vi "纳清_温度校准.vi"(7 "探头":T1(ring), 8 "error in (no error)":errorcluster caption="错误输入（无错误）", 10 "校准温度":sgl, 11 "MB session in":refnum<class "MB_Master.lvclass">) -> (0 "error out":errorcluster caption="错误输出", 3 "MB session out":refnum<class "MB_Master.lvclass">)   [LabVIEW 2016, in "斯坦道多参数.lvlib"]
uses:
  <vilib>/Plasmionique/MB Master/MB_Master/MB_Master.lvclass
  <vilib>/Plasmionique/MB Master/MB Master.lvlib
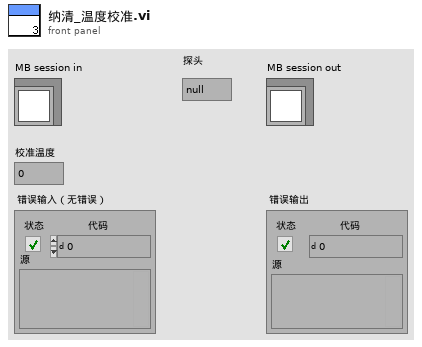
[diagram p1: front panel]
types:
  T1 = enum16{"null", "pH", "DO", "浊度", "电导率", "叶绿素a", "藻密度", "氨氮"}
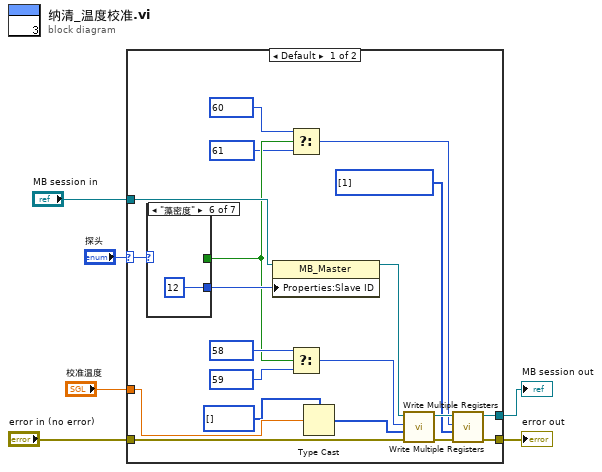
[diagram p0: block diagram]
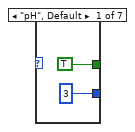
[diagram p2: hidden frame]
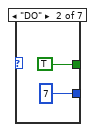
[diagram p3: hidden frame]
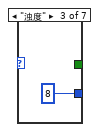
[diagram p4: hidden frame]
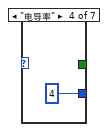
[diagram p5: hidden frame]
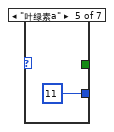
[diagram p6: hidden frame]
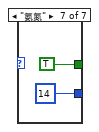
[diagram p7: hidden frame]
diagram:
  n1 = case shown="Default" "探头" {
    selector: "探头" -> [w20 _]
    tunnel: "error in (no error)" -> [w26 w37]
    tunnel: [w17 w37] -> w5
    tunnel: "MB session in" -> [w24 w38]
    tunnel: [w15 w38] -> w3
    tunnel: "校准温度" -> [w22 _]
    frame Default {
      n2 = case shown="\"藻密度\"" w20 {
        tunnel: [3 7 8 4 11 12 14] -> w23
        tunnel: [TRUE TRUE _ _ _ _ TRUE] -> w10
        frame "pH", Default {
        }
        frame "DO" {
        }
        frame "浊度" {
        }
        frame "电导率" {
        }
        frame "叶绿素a" {
        }
        frame "藻密度" {
        }
        frame "氨氮" {
        }
      }
      n3 = property class="MB_Master"(reference=w24, "Properties:Slave ID"=w23) -> (reference out=w25:refnum<class "MB_Master.lvclass">)  [unwired: 1 in, 1 out]
      n4 = Select(t=u16 60 ("starting address"), s=w10, f=u16 61 ("starting address")) -> (s? t:f=w7:u16)
      n5 = Select(t=u16 58 ("starting address"), s=w10, f=u16 59 ("starting address")) -> (s? t:f=w11:u16)
      n6 = Type Cast(type=u16[] [], x=w22) -> (*(type *) &x=w21:u16[])
      n7 = call <vilib>:"Write Multiple Registers.vi"("error in (no error)"=w26, "values"=w21, "starting address"=w11, "MB session in"=w25) -> ("error out"=w18:errorcluster, "MB session out"=w16:refnum<class "MB_Master.lvclass">)  [unwired: 6 in]
      n8 = call <vilib>:"Write Multiple Registers.vi"("error in (no error)"=w18, "values"=u16[] [1], "starting address"=w7, "MB session in"=w16) -> ("error out"=w17:errorcluster, "MB session out"=w15:refnum<class "MB_Master.lvclass">)  [unwired: 6 in]
    }
    frame "null" {
    }
  }
  "error out" <- w5
  "MB session out" <- w3
